vi "All SubFunctions 7.vi"(4 "מק\"ט המכלל":string, 5 "מספר סידורי":string, 7 "מפעיל":string="ANS", 8 "error":errorcluster, 11 "Path for Log":path) -> (0 "error IO":errorcluster)   [LabVIEW 2014]
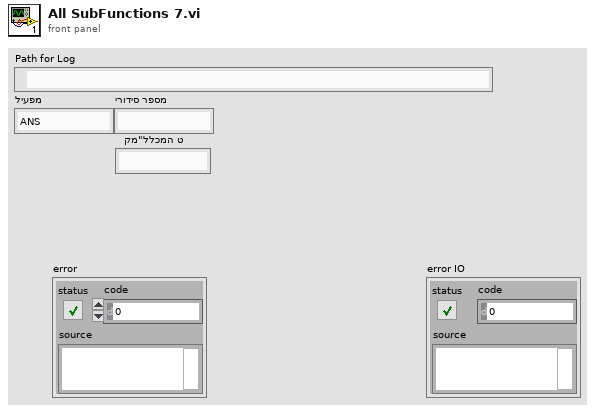
[diagram p1: front panel]
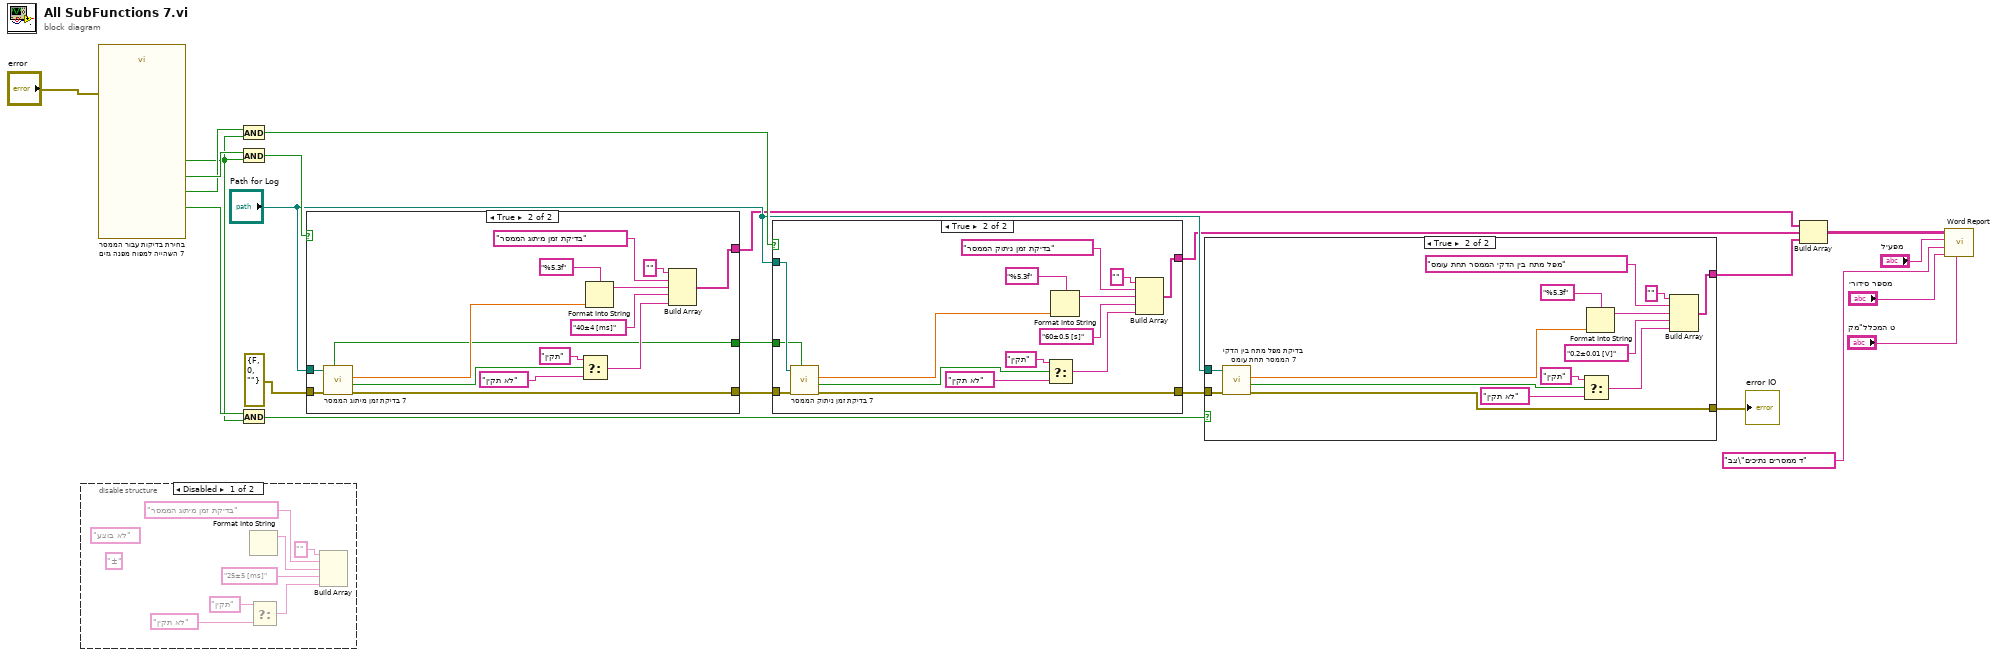
[diagram p0: block diagram]
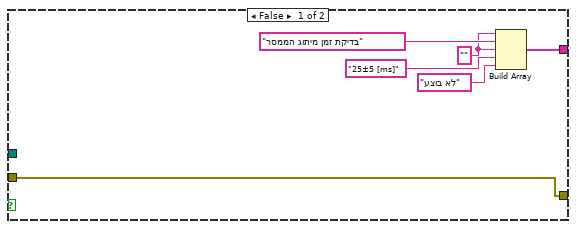
[diagram p3: hidden frame]
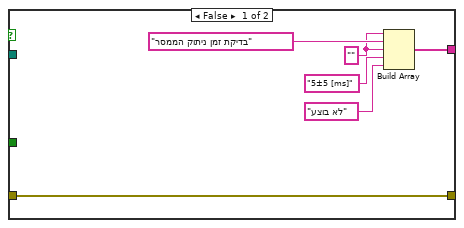
[diagram p4: hidden frame]
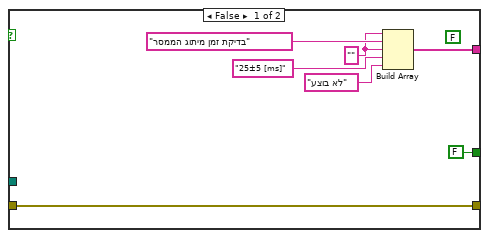
[diagram p5: hidden frame]
diagram:
  n1 = disable-structure shown="Disabled" {
    frame Disabled {
      (unwired) "±"
      (unwired) "לא בוצע"
      n2 = Format Into String() -> (resulting string=w27:string)  [unwired: 4 in, 1 out]
      n3 = Select(t="תקין", f="לא תקין") -> (s? t:f=w29:string)  [unwired: 1 in]
      n4 = Build Array("" ("element"), "בדיקת זמן מיתוג הממסר" ("element"), w27, "25±5 [ms]" ("element"), w29) -> ()  [unwired: 1 out]
    }
    frame Enabled {
    }
  }
  n5 = call "בחירת בדיקות עבור הממסר השהייה למפוח מפנה גזים 7.vi"("error in (no error)"="error") -> ("בדיקת מפל מתח בין דקי הממסר תחת עומס"=w14:bool, "בדיקת זמן ניתוק הממסר"=w16:bool, "בדיקת זמן מיתוג הממסר"=w18:bool, "OK"=w12:bool)  [unwired: 13 in, 2 out]
  n6 = And(x=w16, y=w12) -> (x .and. y?=w15:bool)
  n7 = And(x=w18, y=w12) -> (x .and. y?=w17:bool)
  n8 = And(x=w14, y=w12) -> (x .and. y?=w13:bool)
  n9 = case shown="True" w17 {
    tunnel: [w31 w51] -> w20
    tunnel: "Path for Log" -> [_ w50]
    tunnel: [w32 w40] -> w9
    tunnel: errorcluster {"status"=FALSE, "code"=0, "source"=""} ("error out") -> [w31 w38]
    tunnel: [FALSE ("Userresult") w37] -> w1
    frame False {
      w34 = "" ("element")
      (unwired) FALSE ("resultUserPrompt")
      n10 = Build Array(w34, "בדיקת זמן מיתוג הממסר" ("element"), w34, "25±5 [ms]" ("element"), "לא בוצע") -> (w32:string[])
    }
    frame True {
      n11 = call "בדיקת זמן מיתוג הממסר 7.vi"("error"=w38, "Path for Log"=w50) -> ("error out"=w51:errorcluster, "בטוח כן/לא"=w42:bool, "בדיקת זמן מיתוג הממסר"=w41:dbl, "Userresult"=w37:bool)  [unwired: 6 in]
      n12 = Select(t="תקין", s=w42, f="לא תקין") -> (s? t:f=w43:string)
      n13 = Format Into String(format string="%5.3f", w41) -> (resulting string=w45:string)  [unwired: 2 in, 1 out]
      n14 = Build Array("" ("element"), "בדיקת זמן מיתוג הממסר" ("element"), w45, "40±4 [ms]" ("element"), w43) -> (w40:string[])
    }
  }
  n15 = case shown="True" w15 {
    tunnel: w20 -> [w57 w72]
    tunnel: [w57 w71] -> w19
    tunnel: "Path for Log" -> [_ w70]
    tunnel: [w52 w60] -> w8
    tunnel: w1 -> [_ w58]
    frame False {
      w53 = "" ("element")
      n16 = Build Array(w53, "בדיקת זמן ניתוק הממסר" ("element"), w53, "5±5 [ms]" ("element"), "לא בוצע") -> (w52:string[])
    }
    frame True {
      n17 = call "בדיקת זמן ניתוק הממסר 7.vi"("resultUserPrompt"=w58, "error"=w72, "Path for Log"=w70) -> ("error out"=w71:errorcluster, "בטוח כן/לא"=w61:bool, "בדיקת זמן ניתוק הממסר"=w62:dbl)  [unwired: 6 in]
      n18 = Select(t="תקין", s=w61, f="לא תקין") -> (s? t:f=w63:string)
      n19 = Format Into String(format string="%5.3f", w62) -> (resulting string=w65:string)  [unwired: 2 in, 1 out]
      n20 = Build Array("" ("element"), "בדיקת זמן ניתוק הממסר" ("element"), w65, "60±0.5 [s]" ("element"), w63) -> (w60:string[])
    }
  }
  n21 = case shown="True" w13 {
    tunnel: [w78 w92] -> w21
    tunnel: w19 -> [w78 w91]
    tunnel: "Path for Log" -> [_ w90]
    tunnel: [w73 w80] -> w7
    frame False {
      w74 = "" ("element")
      n22 = Build Array(w74, "בדיקת זמן מיתוג הממסר" ("element"), w74, "25±5 [ms]" ("element"), "לא בוצע") -> (w73:string[])
    }
    frame True {
      n23 = call "בדיקת מפל מתח בין הדקי הממסר תחת עומס 7.vi"("error"=w91, "Path for Log"=w90) -> ("error IO"=w92:errorcluster, "בטווח כן/לא"=w81:bool, "מפל מתח בין דקי הממסר תחת עומס"=w82:dbl)  [unwired: 6 in, 1 out]
      n24 = Select(t="תקין", s=w81, f="לא תקין") -> (s? t:f=w83:string)
      n25 = Format Into String(format string="%5.3f", w82) -> (resulting string=w85:string)  [unwired: 2 in, 1 out]
      n26 = Build Array("" ("element"), "מפל מתח בין הדקי הממסר תחת עומס" ("element"), w85, "0.2±0.01 [V]" ("element"), w83) -> (w80:string[])
    }
  }
  "error IO" <- w21
  n27 = Build Array(w9, w8, w7) -> (w10:string[][])
  n28 = call "Word Report.vi"("מק\"ט המכלל"="מק\"ט המכלל", "מספר סידורי"="מספר סידורי", "שם הצב\"ד"="צב\"ד ממסרים נתיכים", "מפעיל"="מפעיל", "Array"=w10) -> ()  [unwired: 7 in]
